vi "appendix_getTableData.vi"(1 "appended path":path) -> (0 "TableData":T1[](array[typedef]))   [LabVIEW 2016]
uses:
  WorReport_tableData.ctl
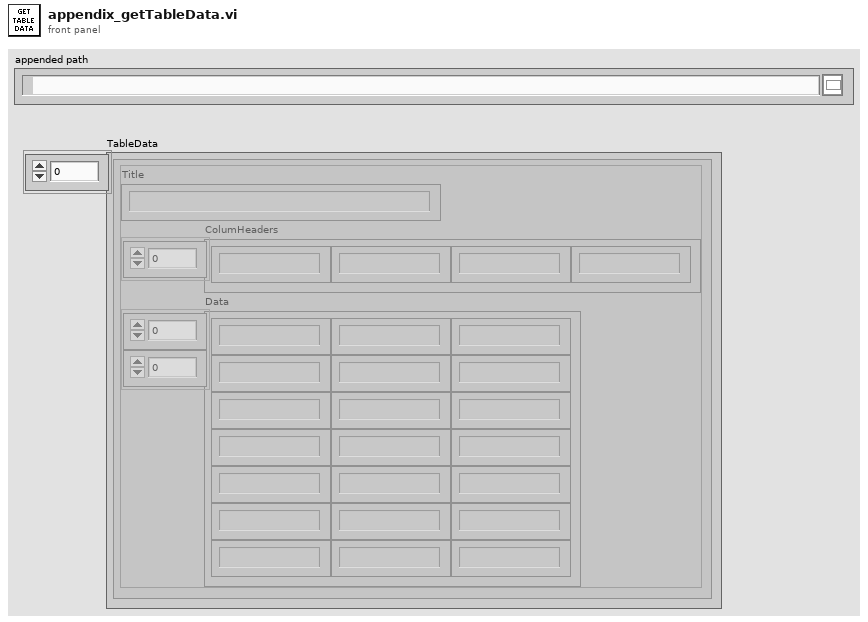
[diagram p1: front panel]
types:
  T1 = typedef "WorReport_tableData.ctl" = cluster{"Title":string, "ColumHeaders":string[], "Data":string[][]}
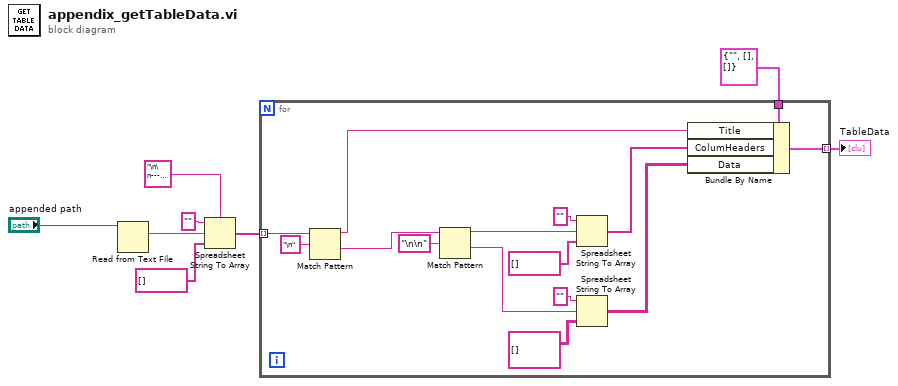
[diagram p0: block diagram]
diagram:
  n1 = Read from Text File(file (use dialog)="appended path") -> (text=w7:string)  [unwired: 3 in, 3 out]
  n2 = Spreadsheet String To Array(delimiter (Tab)="\n\n---   ---   ---   ---   ---   ---   ---   ---   ---   ---   \n\n" ("string"), format string="", spreadsheet string=w7, array type (2D Dbl)=string[] [] ("format string")) -> (array=w3:string[])
  n3 = for {
    tunnel: w3 -> [w23] mode=indexing
    tunnel: T1 {"Title"="", "ColumHeaders"=[], "Data"=[]} ("tableData") -> [w21]
    tunnel: [w14] -> w1 mode=indexing
    n4 = Match Pattern(string=w23, regular expression="\n") -> (before substring=w13:string, after substring=w15:string)  [unwired: 1 in, 2 out]
    n5 = Match Pattern(string=w15, regular expression="\n\n") -> (before substring=w9:string, after substring=w16:string)  [unwired: 1 in, 2 out]
    n6 = Spreadsheet String To Array(format string="", spreadsheet string=w9, array type (2D Dbl)=string[] [] ("format string")) -> (array=w20:string[])  [unwired: 1 in]
    n7 = Spreadsheet String To Array(format string="", spreadsheet string=w16, array type (2D Dbl)=string[][] [] ("format string")) -> (array=w17:string[][])  [unwired: 1 in]
    n8 = Bundle By Name(cluster=w21, "Title"=w13, "ColumHeaders"=w20, "Data"=w17) -> (w14:T1)
  }
  "TableData" <- w1
